vi "U16 Image Data Processing.vi"() -> ()   [LabVIEW 2020, in "examples.lvlib"]
uses:
  examples.lvlib
  image/CLAHE/CLAHE.lvclass
  image/image.lvlib
  image/CLAHE/Apply (U16 Array).vi
  image/Draw Image to Picture (Greyscale).vi
  image/New Image (Greyscale Preallocated).vi
  image/New Image (Greyscale Array).vi
  common/Image Size (Integer).ctl
  common/common.lvlib
panel:
  out "CLAHE":picture caption="(Contrast Limited Adaptive Histogram Equalization)"
  out "Basic Divide":picture
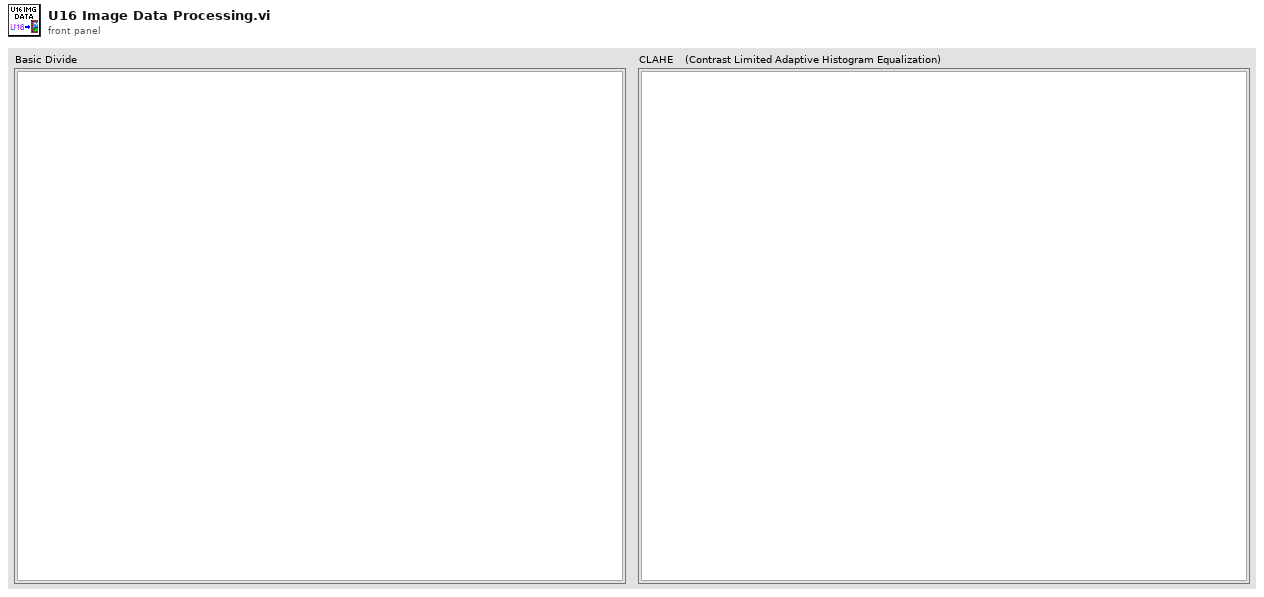
[diagram p1: front panel]
types:
  T1 = typedef "common.lvlib/Image Size (Integer).ctl" = cluster{"Width":u16, "Height":u16}
  T2 = typedef "image.lvlib/Greyscale Image.ctl" = refnum<data-value>
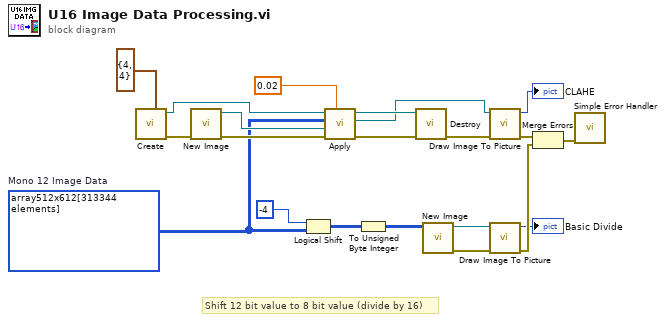
[diagram p0: block diagram]
diagram:
  w4 = u16[][] array512x612[313344 elements]  # Mono 12 Image Data
  # "Shift 12 bit value to 8 bit value (divide by 16)"
  n1 = call "Create.vi"("Grid Size"=T1 {"Width"=4, "Height"=4}) -> ("error out"=w13:errorcluster, "CLAHE"=w21:refnum<class "CLAHE.lvclass">)  [unwired: 9 in]
  n2 = call-poly "New Image.vi"("error in (no error)"=w13) -> ("error out"=w12:errorcluster, "Greyscale Image"=w20:T2)  [unwired: 9 in]
  n3 = Logical Shift(y=i16 -4, x=w4) -> (x << y=w2:u16[][])
  n4 = call-poly "Apply.vi"("Scaling Factor (Default 1.0/256.0)"=0.02, "error in (no error)"=w12, "Destination Image in"=w20, "Mono 16 Image Data"=w4, "CLAHE in"=w21) -> ("error out"=w18:errorcluster, "Destination Image"=w17:T2, "CLAHE"=w19:refnum<class "CLAHE.lvclass">)  [unwired: 4 in]
  n5 = To Unsigned Byte Integer(number=w2) -> (unsigned 8bit integer=w15:u8[][])
  n6 = call "Destroy.vi"("error in (no error)"=w18, "CLAHE"=w19) -> ("error out"=w16:errorcluster)  [unwired: 9 in]
  n7 = call-poly "New Image.vi"("U8 Greyscale Data"=w15) -> ("error out"=w10:errorcluster, "Greyscale Image"=w14:T2)  [unwired: 9 in]
  n8 = call-poly "Draw Image To Picture.vi"("error in (no error)"=w16, "Greyscale Image Source in"=w17) -> ("error out"=w9:errorcluster, "Picture"=→"CLAHE":picture)  [unwired: 8 in]
  n9 = call-poly "Draw Image To Picture.vi"("error in (no error)"=w10, "Greyscale Image Source in"=w14) -> ("error out"=w8:errorcluster, "Picture"=→"Basic Divide":picture)  [unwired: 8 in]
  n10 = Merge Errors(w9, w8) -> (w7:errorcluster)
  n11 = call <vilib>:"Simple Error Handler.vi"("error in (no error)"=w7) -> ()  [unwired: 4 in, 5 out]
